vi "2 RudderControlPI.vi"(9 "use PID?":bool=TRUE, 10 "Desired Heading":dbl) -> (2 "Rudder Output":dbl)   [LabVIEW 2011]
uses:
  2 Typedefs/PI Constants.ctl
  2 Globals/2 Global.vi
  2 Globals/2 TuningConstants.vi
  <vilib>/addons/control/pid/NI_PID_pid.lvlib
  <vilib>/addons/control/pid/pid.llb/PID (DBL).vi
  <vilib>/ptbypt/NI_PtbyPt.lvlib
  <vilib>/addons/control/pid/NI_PID_autopid.lvlib
panel:
  out "PID gains out":T1={"proportional gain (Kc)"=1.0, "integral time (Ti, min)"=0.01, "derivative time (Td, min)"=0.0} {"derivative time (Td, min)" format="%.3f"; "integral time (Ti, min)" format="%.3f"; "proportional gain (Kc)" format="%.3f"}
  out "tuning completed?":bool
  in  "autotuning parameters":T2={"controller type"=1, "relay cycles"=3, "relay amplitude"=1.0, "control specification"=2, "PV noise level"=0.1} {"PV noise level" format="%.2f"; "control specification" items=["normal", "fast", "slow"]; "relay amplitude" format="%.2f"; "controller type" items=["PID", "PI", "P"]}
  in  "autotune? (F)":bool
  out "PID State":dbl format="%0.2f"
  out "PID setpoint":dbl
  out "PI Constants":T3={"Proportional Gain"=5000.0, "Integral Time"=0.2, "Derivative Time"=0.1}
  in  "Maximum Rudder":dbl=40.0
  out "Current Heading":dbl
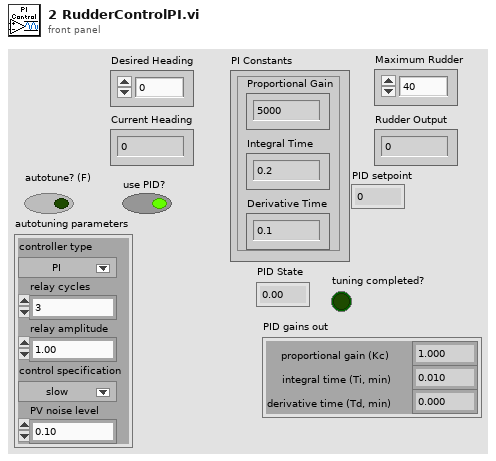
[diagram p1: front panel]
types:
  T1 = cluster{"proportional gain (Kc)":dbl, "integral time (Ti, min)":dbl, "derivative time (Td, min)":dbl}
  T2 = cluster{"controller type":u16, "relay cycles":i32, "relay amplitude":dbl, "control specification":u16, "PV noise level":dbl}
  T3 = typedef "PI Constants.ctl" = cluster{"Proportional Gain":dbl, "Integral Time":dbl, "Derivative Time":dbl}
  T4 = typedef "heading.ctl" = dbl
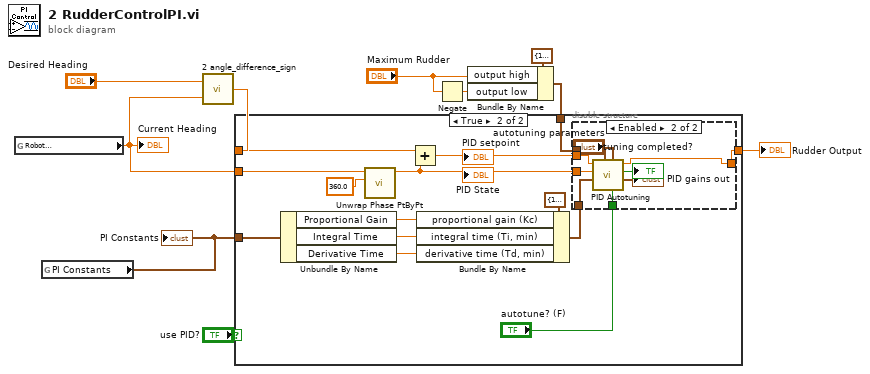
[diagram p0: block diagram]
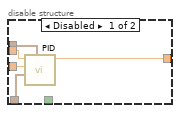
[diagram p3: hidden frame]
diagram:
  n1 = global read "2 Global.vi" "Robot\nHeading"() -> (w3:T4)
  "Current Heading" <- w3
  n2 = global read "2 TuningConstants.vi" "PI Constants"() -> (w1:T3)
  "PI Constants" <- w1
  n3 = call "2 angle_difference_sign.vi"("Angle 2"=w3, "Angle 1"="Desired Heading") -> ("Difference"=w9:dbl)
  n4 = Negate(x="Maximum Rudder") -> (-x=w7:dbl)
  n5 = Bundle By Name(cluster=cluster{"output high":dbl, "output low":dbl} {"output high"=100.0, "output low"=-100.0} ("output range"), "output high"="Maximum Rudder", "output low"=w7) -> (w4:cluster{"output high":dbl, "output low":dbl})
  n6 = case shown="True" "use PID?" {
    tunnel: w9 -> [w11 w16]
    tunnel: w1 -> [_ w23]
    tunnel: w4 -> [_ w25]
    tunnel: w3 -> [_ w17]
    tunnel: [w11 w13] -> w2
    frame False {
    }
    frame True {
      n7 = Unbundle By Name(w23) -> ("Proportional Gain"=w21:dbl, "Integral Time"=w20:dbl, "Derivative Time"=w19:dbl)
      n8 = call <vilib>:"Unwrap Phase PtByPt.vi"("wrap base"=360.0, "phase"=w17) -> ("unwrapped phase"=w15:dbl)  [unwired: 9 in]
      "PID State" <- w15
      n9 = Add(x=w16, y=w15) -> (x+y=w14:dbl)
      "PID setpoint" <- w14
      n10 = Bundle By Name(cluster=T1 {"proportional gain (Kc)"=1.0, "integral time (Ti, min)"=0.01, "derivative time (Td, min)"=0.0} ("PID gains"), "proportional gain (Kc)"=w21, "integral time (Ti, min)"=w20, "derivative time (Td, min)"=w19) -> (w22:T1)
      n11 = disable-structure shown="Enabled" {
        disable-tunnel: w25 -> [w30 w35]
        disable-tunnel: w22 -> [w29 w37]
        disable-tunnel: w15 -> [w28 w38]
        disable-tunnel: w14 -> [w27 w39]
        disable-tunnel: [w26 w31] -> w13
        disable-tunnel: "autotune? (F)" -> [_ w36]
        frame Disabled {
          n12 = call-poly <vilib>:"PID.vi"("output range"=w30, "PID gains"=w29, "process variable"=w28, "setpoint"=w27) -> ("output"=w26:dbl)  [unwired: 6 in, 1 out]
        }
        frame Enabled {
          n13 = call <vilib>:"PID Autotuning.vi"("autotune? (F)"=w36, "autotuning parameters"="autotuning parameters", "output range"=w35, "PID gains"=w37, "process variable"=w38, "setpoint"=w39) -> ("PID gains out"=→"PID gains out":T1, "tuning completed?"=→"tuning completed?":bool, "output"=w31:dbl)  [unwired: 2 in, 1 out]
        }
      }
    }
  }
  "Rudder Output" <- w2
